vi "Actor Core.vi"(8 "error in":errorcluster, 11 "Analyze Actor in":refnum<class "Analyze Actor.lvclass">) -> (0 "error out":errorcluster, 3 "Actor out":refnum<class "Actor.lvclass">)   [LabVIEW 2014, in "Analyze Actor.lvlib" / "Analyze Actor.lvclass"]
doc: "(<B>Filename</B>: Actor Framework.lvlib:Actor.lvclass:Actor Core.vi)\n\nReceives messages to the actor, reacts to them, and initiates any error handling that may shut the actor down.\n\nDescendant classes may override this VI to append parallel tasks for the actor to complete while it handles messages. Overrides use the Call Parent Method node."
uses:
  Analyze Actor.lvclass
  <vilib>/ActorFramework/Actor/Actor.lvclass
  HIJ Vision Display/HIJ Vision Display/Analyze.ctl
  <vilib>/vision/Image Controls.llb/IMAQ Image.ctl
  Analyze Classes/Analyze BaseClass/Analyze BaseClass/Analyze BaseClass.lvclass
  Abstract Messages/Publish Analyze Results Msg/Publish Analyze Results Msg.lvclass
  Results and Overlays/Results Base/Analyze Results Base.lvclass
  Analyze Actor.lvclass/Analyze Actor.ctl
  <vilib>/ActorFramework/Actor/Actor.lvclass/Actor.ctl
  <vilib>/ActorFramework/Message Enqueuer/Message Enqueuer.lvclass/Message Enqueuer.ctl
  <vilib>/ActorFramework/Report Error Msg/Report Error Msg.lvclass/Report Error Msg.ctl
  <vilib>/ActorFramework/Message Enqueuer/Init from Existing Queue.vi
  <vilib>/ActorFramework/Message Enqueuer/Enqueue.vi
  <vilib>/ActorFramework/Message Priority Queue/Priority Enqueue.vi
  <vilib>/ActorFramework/Message Enqueuer/Message Enqueuer.lvclass
  <vilib>/ActorFramework/Report Error Msg/Report Error Msg.lvclass
panel:
  in  "StopSignal":bool=TRUE
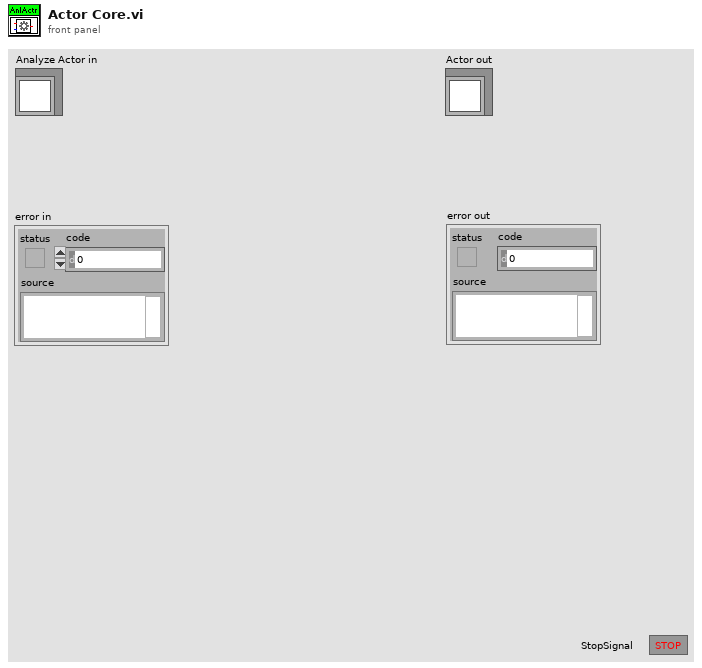
[diagram p1: front panel]
types:
  T1 = typedef "Analyze Actor.lvlib/Analyze Actor.lvclass/Analyze.ctl" = cluster{"Image":T2, "ImageNr":i32, "Analyze Objects":refnum<class "Analyze BaseClass.lvclass">[], "Publish Analyze Results Msg":refnum<class "Publish Analyze Results Msg.lvclass">, "Pre Results":refnum<class "Analyze Results Base.lvclass">[]}
  T2 = typedef "IMAQ Image.ctl" = refnum<image>
  T3 = typedef "Image Type" = u32
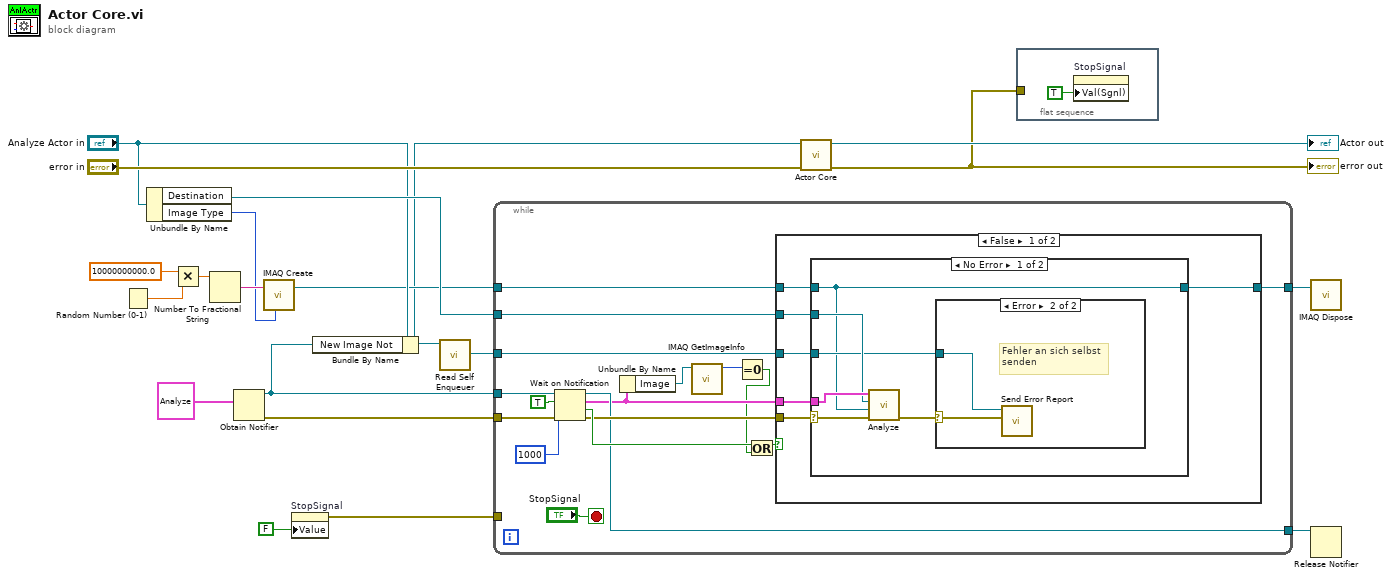
[diagram p0: block diagram]
diagram:
  n1 = Random Number (0-1)() -> (number: 0 to 1=w10:dbl)
  n2 = Unbundle By Name("Analyze Actor in") -> ("Destination"=w20:refnum<class "Message Enqueuer.lvclass">, "Image Type"=w6:T3)
  n3 = Multiply(x=10000000000.0, y=w10) -> (x*y=w9:dbl)
  n4 = Number To Fractional String(number=w9) -> (F-format string=w8:string)  [unwired: 3 in]
  n5 = Obtain Notifier(notification data type=T1 {"Image"=refnum, "ImageNr"=0, "Analyze Objects"=[], "Publish Analyze Results Msg"=refnum, "Pre Results"=[]}) -> (notifier out=w11:refnum<notifier>, error out=w16:errorcluster)  [unwired: 3 in, 1 out]
  n6 = call "IMAQ Create"("Image Name"=w8, "Image Type"=w6) -> ("New Image"=w5:T2)  [unwired: 3 in, 1 out]
  n7 = property on="StopSignal" class="Bool (strict)"("Value"=FALSE ("Value (Signaling)")) -> (error out=w17:errorcluster)  [unwired: 2 in, 1 out]
  n8 = Bundle By Name(cluster="Analyze Actor in", "New Image Not"=w11) -> (w2:refnum<class "Analyze Actor.lvclass">)
  n9 = call <vilib>:"Read Self Enqueuer.vi"("Actor"=w2) -> ("Self Enqueuer"=w1:refnum<class "Message Enqueuer.lvclass">)  [unwired: 10 in]
  n10 = while {
    tunnel: w11 -> [w30]
    tunnel: w16 -> [w37]
    tunnel: w17 -> [_]
    tunnel: w1 -> [w35]
    tunnel: [w29] -> w14
    tunnel: w20 -> [w28]
    tunnel: w5 -> [w27]
    tunnel: [w26] -> w4
    stop <- "StopSignal" stop-if-true
    n11 = Wait on Notification(notifier=w30, ignore previous (F)=TRUE, timeout in ms (-1)=1000, error in (no error)=w37) -> (notifier out=w29:refnum<notifier>, notification=w25:T1, timed out?=w34:bool, error out=w31:errorcluster)
    n12 = Unbundle By Name(w25) -> ("Image"=w24:T2)
    n13 = call "IMAQ GetImageInfo"("Image"=w24) -> ("X Resolution"=w23:i32)  [unwired: 3 in, 7 out]
    n14 = Equal To 0?(x=w23) -> (x = 0?=w21:bool)
    n15 = Or(x=w34, y=w21) -> (x .or. y?=w22:bool)
    n16 = case shown="False" w22 {
      tunnel: w25 -> [w42 _]
      tunnel: w35 -> [w41 _]
      tunnel: w31 -> [w43 _]
      tunnel: w28 -> [w40 _]
      tunnel: w27 -> [w39 w53]
      tunnel: [w38 w53] -> w26
      frame False {
        n17 = case shown="No Error" w43 {
          selector: w43 -> [w48 _]
          tunnel: w42 -> [w49 _]
          tunnel: w41 -> [w45 _]
          tunnel: w40 -> [w46 _]
          tunnel: w39 -> [w44 w52]
          tunnel: [w44 w52] -> w38
          frame No Error {
            n18 = call "Analyze.vi"("error in (no error)"=w48, "Work Image"=w44, "Destination"=w46, "Analyze Data"=w49) -> ("error out"=w47:errorcluster)  [unwired: 7 in]
            n19 = case shown="Error" w47 {
              selector: w47 -> [_ w51]
              tunnel: w45 -> [_ w50]
              frame No Error {
              }
              frame Error {
                # "Fehler an sich selbst\nsenden"
                n20 = call <vilib>:"Send Error Report.vi"("Error From Sender"=w51, "Message Enqueuer"=w50) -> ()  [unwired: 9 in, 1 out]
              }
            }
          }
          frame Error {
          }
        }
      }
      frame True {
      }
    }
  }
  n21 = call-parent "Actor Core.vi"("error in"="error in", "Actor in"=w2) -> ("error out"=w13:errorcluster, "Actor out"=→"Actor out":refnum<class "Actor.lvclass">)  [unwired: 8 in]
  "error out" <- w13
  n22 = flat-sequence {
    tunnel: w13 -> [_]
    frame #0 {
      n23 = property on="StopSignal" class="Bool (strict)"("Val(Sgnl)"=TRUE ("Value (Signaling)")) -> ()  [unwired: 2 in, 2 out]
    }
  }
  n24 = call "IMAQ Dispose"("Image"=w4) -> ()  [unwired: 5 in, 1 out]
  n25 = Release Notifier(notifier=w14) -> ()  [unwired: 2 in, 3 out]
